vi "ET_Testing.vi"() -> ()   [LabVIEW 2020]
uses:
  Set Time.vi
  Global Variables/Training_Status.vi
  Global Variables/Global Enable Logging.vi
  Global Variables/Trial_Flag.vi
  Global Variables/Time_Trigger.vi
  Global Variables/Global Label.vi
  Global Variables/Global Send To ANN.vi
panel:
  out "SYSTEM HISTOGRAM ET":T1(graph)
  out "Statistical Metrics System":T2
  out "Sample index":u32
  out "System Mode":enum16{"Training", "Classifying"}(ring)
  out "Continuous Plot SS":dbl[](graph)
  out "Statistical Metrics Sample":T2
  out "SAMPLE HISTOGRAM ET":T1(graph)
  out "ET History":dbl[](array[numeric])
  in  "Stop ET Measurement":bool
  # "Currently, 5400"
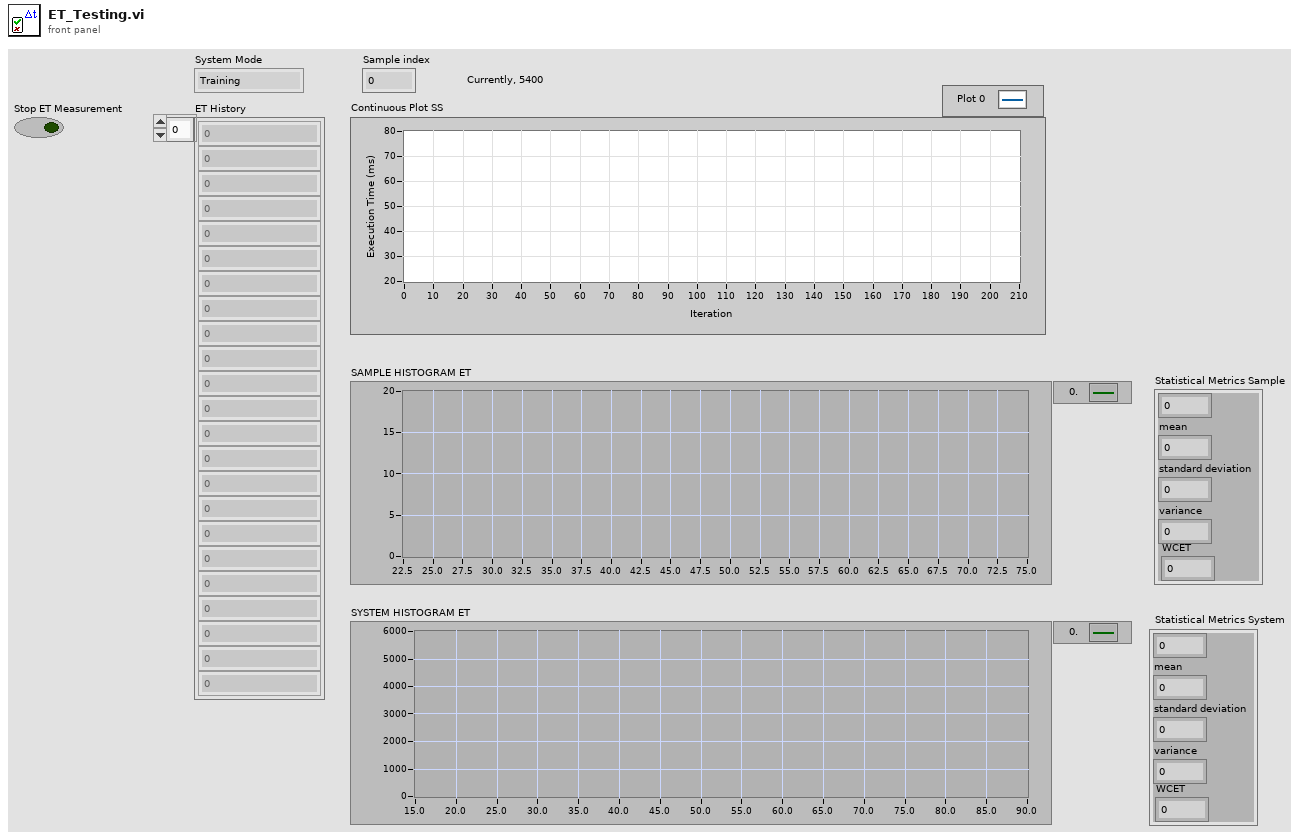
[diagram p1: front panel]
types:
  T1 = cluster{"X Values":dbl[], "Histogram: h(x)":i32[]}
  T2 = cluster{dbl, "mean":dbl, "standard deviation":dbl, "variance":dbl, "WCET":dbl}
  T3 = enum16{"open", "replace", "create", "open or create", "replace or create", "replace or create with confirmation"}
  T4 = cluster{dbl, "mean":dbl, "standard deviation":dbl, "variance":dbl, dbl}
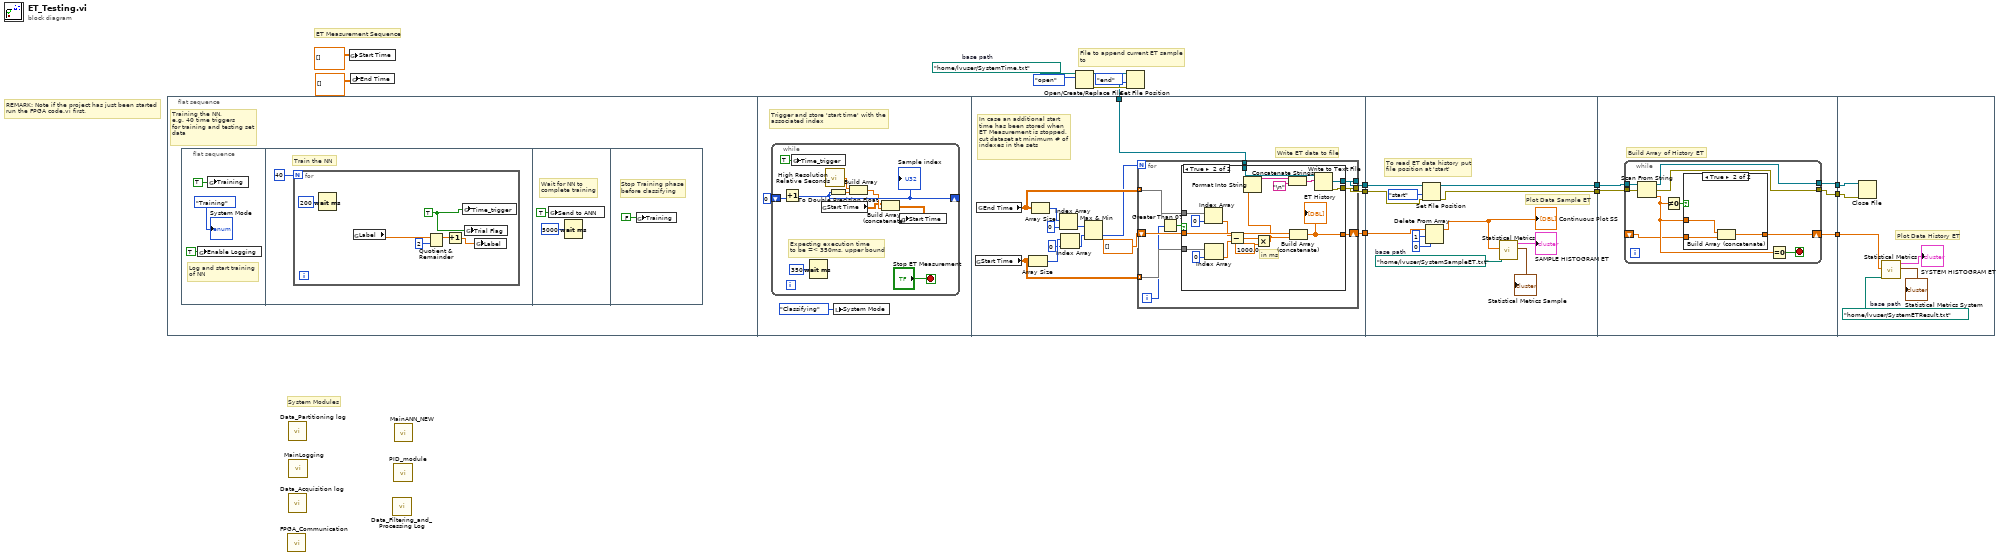
[diagram p0: block diagram]
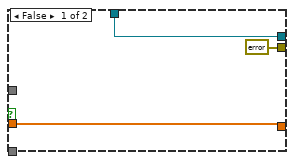
[diagram p2: hidden frame]
diagram:
  w14 = path "/home/lvuser/SystemTime.txt"  # base path
  # "File to append current ET sample \nto"
  # "REMARK: Note if the project has just been started\nrun the FPGA code.vi first."
  # "System Modules"
  # "ET Measurement Sequence"
  n1 = flat-sequence {
    tunnel: w9 -> [w44]
    tunnel: [w45] -> w8
    tunnel: [w43] -> w7
    tunnel: [w42] -> w6
    tunnel: w8 -> [w88]
    tunnel: w7 -> [w93]
    tunnel: w6 -> [w91]
    tunnel: [w89] -> w5
    tunnel: [w90] -> w4
    tunnel: w5 -> [w100]
    tunnel: w4 -> [w101]
    tunnel: [w97] -> w3
    tunnel: [w99] -> w2
    tunnel: [w98] -> w1
    tunnel: w3 -> [w115]
    tunnel: w2 -> [w119]
    tunnel: w1 -> [w116]
    frame #0 {
      # "Training the NN, \ne.g. 40 time triggers \nfor training and testing set \ndata"
      n2 = flat-sequence {
        frame #0 {
          # "Log and start training \nof NN"
          n3 = global write "Global Enable Logging.vi" "Enable Logging"(TRUE ("Enable Logging")) -> ()
          n4 = global write "Training_Status.vi" "Training"(TRUE ("Training")) -> ()
          "System Mode" <- enum16{"Training", "Classifying"}."Training" ("System Mode")
        }
        frame #1 {
          # "Train the NN"
          n5 = for {
            N: 40 -> [_]
            w22 = TRUE
            n6 = Wait (ms)(milliseconds to wait=u32 200) -> ()  [unwired: 1 out]
            n7 = global read "Global Label.vi" "Label"() -> (w24:dbl)
            n8 = Quotient & Remainder(x=w24, y=u8 2) -> (x-y*floor(x/y)=w23:dbl)  [unwired: 1 out]
            n9 = Increment(x=w23) -> (x+1=w25:dbl)
            n10 = global write "Time_Trigger.vi" "Time_trigger"(w22) -> ()
            n11 = global write "Trial_Flag.vi" "Trial Flag"(w22) -> ()
            n12 = global write "Global Label.vi" "Label"(w25) -> ()
          }
        }
        frame #2 {
          # "Wait for NN to \ncomplete training"
          n13 = global write "Global Send To ANN.vi" "Send to ANN"(TRUE ("Send to ANN")) -> ()
          n14 = Wait (ms)(milliseconds to wait=u32 5000) -> ()  [unwired: 1 out]
        }
        frame #3 {
          # "Stop Training phase \nbefore classifying"
          n15 = global write "Training_Status.vi" "Training"(FALSE ("Training")) -> ()
        }
      }
    }
    frame #1 {
      # "Trigger and store 'start time' with the \nassociated index"
      n16 = while {
        shift-right: [w41] -> _
        shift-left: u32 0 ("milliseconds to wait") -> [w37]
        stop <- "Stop ET Measurement" stop-if-true
        # "Expecting execution time \nto be =< 350ms, upper bound"
        n17 = Increment(x=w37) -> (x+1=w41:u32)
        "Sample index" <- w41
        n18 = global write "Time_Trigger.vi" "Time_trigger"(TRUE ("Time Triger")) -> ()
        n19 = Wait (ms)(milliseconds to wait=u32 350) -> ()  [unwired: 1 out]
        n20 = global read "Set Time.vi" "Start Time"() -> (w33:dbl[][])
        n21 = call <vilib>:"High Resolution Relative Seconds.vi"() -> ("relative seconds"=w32:dbl)
        n22 = To Double Precision Float(number=w41) -> (double precision float=w35:dbl)
        n23 = Build Array(w32, w35) -> (w34:dbl[])
        n24 = Build Array (concatenate)(w33, w34) -> (w36:dbl[][])
        n25 = global write "Set Time.vi" "Start Time"(w36) -> ()
      }
      n26 = local write "System Mode"(enum16{"Training", "Classifying"}."Classifying" ("System Mode")) -> ()
    }
    frame #2 {
      # "Write ET data to file"
      # "In case an additional start\ntime has been stored when \nET Measurement is stopped, \ncut dataset at minimum # of \nindexes in the sets"
      n27 = global read "Set Time.vi" "Start Time"() -> (w49:dbl[][])
      n28 = global read "Set Time.vi" "End Time"() -> (w48:dbl[][])
      n29 = Array Size(array=w49) -> (size(s)=w53:i32[])
      n30 = Array Size(array=w48) -> (size(s)=w55:i32[])
      n31 = Index Array(array=w55, index=0) -> (element=w51:i32)
      n32 = Index Array(array=w53, index=0) -> (element=w50:i32)
      n33 = Max & Min(x=w51, y=w50) -> (min(x,y)=w46:i32)  [unwired: 1 out]
      n34 = for {
        N: w46 -> [_]
        tunnel: w49 -> [w63] mode=indexing
        tunnel: w48 -> [w64] mode=indexing
        shift-right: [w62] -> w45
        shift-left: dbl[] [] -> [w61]
        tunnel: w44 -> [w60]
        tunnel: [w59] -> w43
        tunnel: [w58] -> w42
        i -> [w56]
        n35 = Greater Than 0?(x=w56) -> (x > 0?=w57:bool)
        n36 = case shown="True" w57 {
          tunnel: w64 -> [_ w84]
          tunnel: w63 -> [_ w83]
          tunnel: [w65 w82] -> w62
          tunnel: w61 -> [w65 w81]
          tunnel: w60 -> [w67 w80]
          tunnel: [w67 w79] -> w59
          tunnel: [errorcluster {"status"=FALSE, "code"=0, "source"=""} ("error out") w78] -> w58
          frame False {
          }
          frame True {
            # "in ms"
            n37 = Index Array(array=w84, index=0) -> (element=w75:dbl)
            n38 = Index Array(array=w83, index=0) -> (element=w74:dbl)
            n39 = Subtract(x=w75, y=w74) -> (x-y=w73:dbl)
            n40 = Multiply(x=w73, y=1000.0) -> (x*y=w71:dbl)
            n41 = Format Into String(w71) -> (resulting string=w68:string)  [unwired: 3 in, 1 out]
            n42 = Concatenate Strings(w68, "\n") -> (w70:string)
            n43 = Build Array (concatenate)(w81, w71) -> (w82:dbl[])
            "ET History" <- w82
            n44 = Write to Text File(file (use dialog)=w80, text=w70) -> (refnum out=w79:refnum<file>, error out=w78:errorcluster)  [unwired: 2 in, 1 out]
          }
        }
      }
    }
    frame #3 {
      w94 = path "/home/lvuser/SystemSampleET.txt"  # base path
      # "Plot Data Sample ET"
      # "To read ET data history put \nfile position at 'start'"
      n45 = Set File Position(refnum=w93, from (0:start)=enum16{"start", "end", "current"}."start", error in=w91) -> (refnum out=w89:refnum<file>, error out=w90:errorcluster)  [unwired: 1 in]
      n46 = Delete From Array(array=w88, length=1, index=0) -> (array with subset deleted=w87:dbl[])  [unwired: 1 out]
      "Continuous Plot SS" <- w87
      n47 = call "Statistical Metrics.vi"("ET Array"=w87, "base path"=w94) -> ("Histogram Graph"=→"SAMPLE HISTOGRAM ET":T1, "Statistical Metrics"=→"Statistical Metrics Sample":T4)  [unwired: 6 in, 1 out]
    }
    frame #4 {
      # "Build Array of History ET"
      n48 = while {
        tunnel: w100 -> [w110]
        tunnel: w101 -> [w109]
        shift-right: [w105] -> w99
        shift-left: _ -> [w104]
        tunnel: [w103] -> w98
        tunnel: [w102] -> w97
        stop <- w108 stop-if-true
        n49 = Scan From String(w110, w109) -> (w102:refnum<file>, w103:errorcluster, output 1=w106:dbl)  [unwired: 2 in]
        n50 = Not Equal To 0?(x=w106) -> (x != 0?=w107:bool)
        n51 = case shown="True" w107 {
          tunnel: w106 -> [_ w113]
          tunnel: [w111 w114] -> w105
          tunnel: w104 -> [w111 w112]
          frame False {
          }
          frame True {
            n52 = Build Array (concatenate)(w113, w112) -> (w114:dbl[])
          }
        }
        n53 = Equal To 0?(x=w106) -> (x = 0?=w108:bool)
      }
    }
    frame #5 {
      w120 = path "/home/lvuser/SystemETResult.txt"  # base path
      # "Plot Data History ET"
      n54 = Close File(refnum=w115, error in=w116) -> ()  [unwired: 2 out]
      n55 = call "Statistical Metrics.vi"("ET Array"=w119, "base path"=w120) -> ("Histogram Graph"=→"SYSTEM HISTOGRAM ET":T1, "Statistical Metrics"=→"Statistical Metrics System":T4)  [unwired: 6 in, 1 out]
    }
  }
  n56 = call "FPGA_Communication.vi"() -> ()  [unwired: 12 in]
  n57 = call "Data_Partitioning log.vi"() -> ()  [unwired: 11 in]
  n58 = call "Data_Acquisition log.vi"() -> ()  [unwired: 9 in]
  n59 = call "MainLogging.vi"() -> ()  [unwired: 7 in]
  n60 = global write "Set Time.vi" "Start Time"(dbl[][] []) -> ()
  n61 = global write "Set Time.vi" "End Time"(dbl[][] []) -> ()
  n62 = call "Data_Filtering_and_Processing Log.vi"() -> ()  [unwired: 11 in]
  n63 = call "PID_module.vi"() -> ()  [unwired: 11 in]
  n64 = call "MainANN_NEW.vi"() -> ()  [unwired: 12 in]
  n65 = Open/Create/Replace File(file path (use dialog)=w14, operation (0:open)=T3."open") -> (refnum out=w12:refnum<file>, error out=w11:errorcluster)  [unwired: 4 in, 1 out]
  n66 = Set File Position(refnum=w12, from (0:start)=enum16{"start", "end", "current"}."end", error in=w11) -> (refnum out=w9:refnum<file>)  [unwired: 1 in, 1 out]
